vi "Find Control in VI.vi"(8 "error in (no error)":errorcluster, 10 "control label":string, 11 "vi reference in":refnum<vi>) -> (0 "error out":errorcluster, 2 "control reference":refnum<vi>, 3 "vi reference out":refnum<vi>)   [LabVIEW 2015, in "PL Utility.lvlib"]
doc: "Finds control with a specified <b>control label</b> in the VI specified by <b>vi reference</b> and returns <b>control reference</b>."
uses:
  PL Utility.lvlib
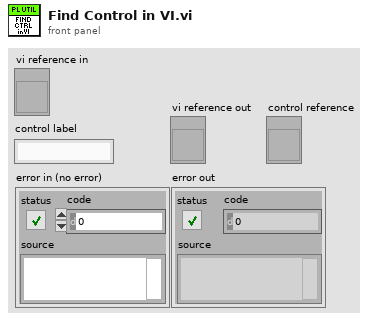
[diagram p1: front panel]
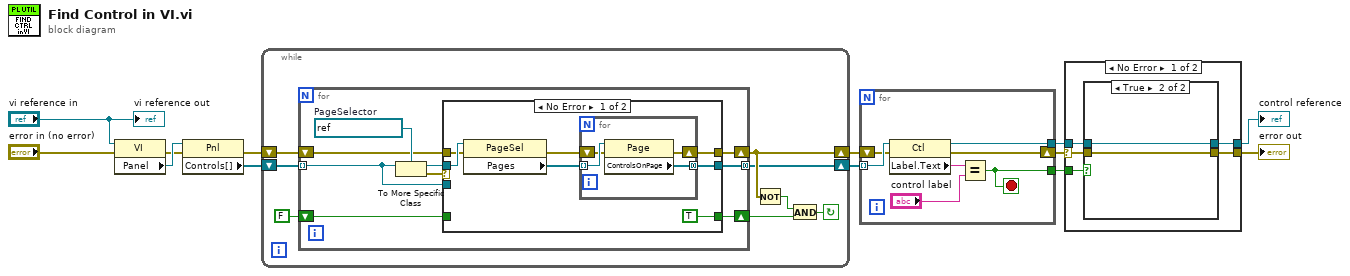
[diagram p0: block diagram]
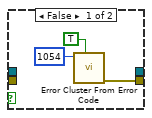
[diagram p2: hidden frame]
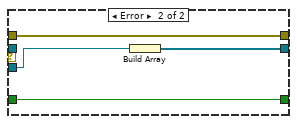
[diagram p4: hidden frame]
diagram:
  n1 = property class="VI"(reference="vi reference in", error in="error in (no error)") -> (error out=w12:errorcluster, "Panel"=w13:refnum<vi>)  [unwired: 1 out]
  n2 = property class="Pnl"(reference=w13, error in=w12) -> (error out=w9:errorcluster, "Controls[]"=w10:refnum<vi>[])  [unwired: 1 out]
  n3 = while {
    shift-right: [w15] -> w8
    shift-left: w9 -> [w20]
    shift-right: [w14] -> w7
    shift-left: w10 -> [w21]
    stop <- w16 continue-if-true
    n4 = for {
      tunnel: w21 -> [w24] mode=indexing
      shift-right: [w25] -> w15
      shift-left: w20 -> [w27]
      tunnel: [w26] -> w14 mode=concatenating
      shift-right: [w23] -> w17
      shift-left: FALSE -> [w22]
      w30 = refnum<vi> refnum  # PageSelector
      n5 = To More Specific Class(target class=w30, reference=w24) -> (specific class reference=w28:refnum<vi>, error out=w29:errorcluster)  [unwired: 1 in]
      n6 = case shown="No Error" w29 {
        tunnel: w28 -> [w37 _]
        tunnel: w27 -> [w36 w45]
        tunnel: [w33 w44] -> w26
        tunnel: [w32 w45] -> w25
        tunnel: w24 -> [_ w43]
        tunnel: [TRUE w42] -> w23
        tunnel: w22 -> [_ w42]
        frame No Error {
          n7 = property class="PageSel"(reference=w37, error in=w36) -> (error out=w34:errorcluster, "Pages"=w35:refnum<vi>[])  [unwired: 1 out]
          n8 = for {
            tunnel: w35 -> [w41] mode=indexing
            shift-right: [w38] -> w32
            shift-left: w34 -> [w40]
            tunnel: [w39] -> w33 mode=concatenating
            n9 = property class="Page"(reference=w41, error in=w40) -> (error out=w38:errorcluster, "ControlsOnPage"=w39:refnum<vi>[])  [unwired: 1 out]
          }
        }
        frame Error {
          n10 = Build Array(w43) -> (w44:refnum<vi>[])
        }
      }
    }
    n11 = Not(x=w15) -> (.not. x?=w18:bool)
    n12 = And(x=w18, y=w17) -> (x .and. y?=w16:bool)
  }
  n13 = for {
    tunnel: w7 -> [w52] mode=indexing
    shift-right: [w50] -> w3
    shift-left: w8 -> [w51]
    tunnel: [w47] -> w1
    tunnel: [w46] -> w2
    stop <- w46 stop-if-true
    n14 = property class="Ctl"(reference=w52, error in=w51) -> (reference out=w47:refnum<vi>, error out=w50:errorcluster, "Label.Text"=w49:string)
    n15 = Equal?(x=w49, y="control label") -> (x = y?=w46:bool)
  }
  n16 = case shown="No Error" w3 {
    selector: w3 -> [w55 w63]
    tunnel: [w56 w63] -> w6
    tunnel: w2 -> [w57 _]
    tunnel: w1 -> [w54 _]
    tunnel: [w53 _] -> w4
    frame No Error {
      n17 = case shown="True" w57 {
        tunnel: [w58 w62] -> w56
        tunnel: w55 -> [_ w62]
        tunnel: w54 -> [_ w61]
        tunnel: [_ w61] -> w53
        frame False {
          n18 = call <vilib>:"Error Cluster From Error Code.vi"("show call chain? (False)"=TRUE, "error code (0)"=1054) -> ("error out"=w58:errorcluster)  [unwired: 7 in]
        }
        frame True {
        }
      }
    }
    frame Error {
    }
  }
  "error out" <- w6
  "control reference" <- w4
  "vi reference out" <- "vi reference in"
